vi "Extract_Channels_From_ITX.vi"(8 "error in":errorcluster, 11 "itx file, N 1d channels":path=path "P:/sample/GaAs/GaAs quantum dots/2008/PL Map/A1 735/060731ASBA_A1_6.0.itx") -> (0 "error out":errorcluster, 1 "wave names":string[](array[string]), 2 "base wavenames":string[](array[string]), 3 "Arr of 1D channels":dbl[][](array[numeric]), 4 "Notes":string)   [LabVIEW 2016]
uses:
  <userlib>/LevyLab/LV to ITX/Data.ITX/Data.ITX.lvclass
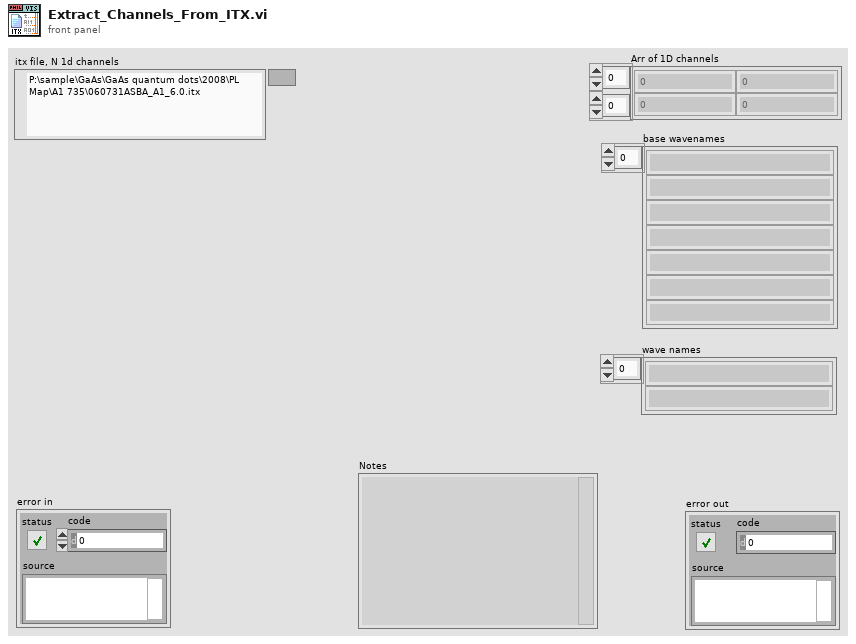
[diagram p1: front panel]
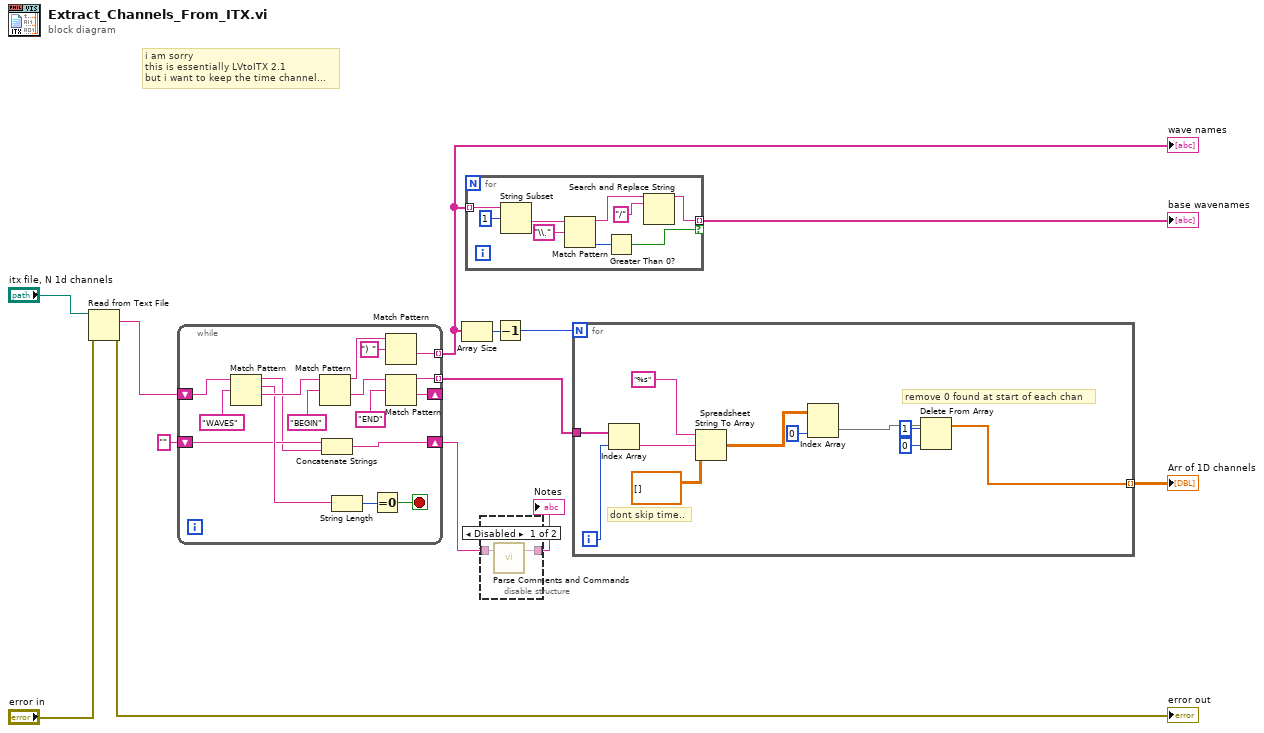
[diagram p0: block diagram]
diagram:
  # "i am sorry \nthis is essentially LVtoITX 2.1\nbut i want to keep the time channel..."
  n1 = Read from Text File(file (use dialog)="itx file, N 1d channels", error in="error in") -> (text=w6:string, error out=→"error out":errorcluster)  [unwired: 1 in, 3 out]
  n2 = while {
    tunnel: [w27] -> w12 mode=indexing
    shift-right: [w28] -> _
    shift-left: w6 -> [w15]
    tunnel: [w23] -> w8 mode=indexing
    shift-right: [w18] -> w11
    shift-left: "" ("regular expression") -> [w17]
    stop <- w24 stop-if-true
    n3 = Match Pattern(string=w15, regular expression="WAVES") -> (before substring=w16:string, match substring=w26:string, after substring=w30:string)  [unwired: 2 out]
    n4 = Match Pattern(string=w30, regular expression="BEGIN" ("regular expression 2")) -> (before substring=w14:string, after substring=w29:string)  [unwired: 3 out]
    n5 = Concatenate Strings(w17, w16) -> (w18:string)
    n6 = String Length(string=w26) -> (length=w25:i32)
    n7 = Equal To 0?(x=w25) -> (x = 0?=w24:bool)
    n8 = Match Pattern(string=w14, regular expression=") ") -> (after substring=w23:string)  [unwired: 4 out]
    n9 = Match Pattern(string=w29, regular expression="END" ("regular expression 3")) -> (before substring=w27:string, after substring=w28:string)  [unwired: 3 out]
  }
  "wave names" <- w8
  n10 = Array Size(array=w8) -> (size(s)=w9:i32)
  n11 = for {
    tunnel: w8 -> [w38] mode=indexing
    tunnel: [w31] -> w5 mode=indexing if=w34
    n12 = String Subset(string=w38, offset (0)=1) -> (substring=w37:string)  [unwired: 1 in]
    n13 = Match Pattern(string=w37, regular expression="\\.") -> (before substring=w32:string, offset past match=w35:i32)  [unwired: 1 in, 2 out]
    n14 = Greater Than 0?(x=w35) -> (x > 0?=w34:bool)
    n15 = Search and Replace String(input string=w32, search string="/") -> (result string=w31:string)  [unwired: 6 in, 3 out]
  }
  "base wavenames" <- w5
  n16 = disable-structure shown="Disabled" {
    disable-tunnel: w11 -> [w41 _]
    disable-tunnel: [w40 _] -> w10
    frame Disabled {
      n17 = call <userlib>:"Parse Comments and Commands.vi"("ITX Notes and Commands"=w41) -> ("Notes"=w40:string)  [unwired: 1 in, 1 out]
    }
    frame Enabled {
    }
  }
  "Notes" <- w10
  n18 = Decrement(x=w9) -> (x-1=w3:i32)
  n19 = for {
    N: w3 -> [_]
    tunnel: w12 -> [w52]
    tunnel: [w43] -> w4 mode=indexing
    i -> [w50]
    # "remove 0 found at start of each chan"
    # "dont skip time.."
    n20 = Index Array(array=w52, index=w50) -> (element=w51:string)
    n21 = Spreadsheet String To Array(format string="%s", spreadsheet string=w51, array type (2D Dbl)=dbl[][] []) -> (array=w48:dbl[][])  [unwired: 1 out]
    n22 = Index Array(array=w48, index (col)=0 ("disabled index (col)")) -> (element=w44:dbl[])  [unwired: 1 in]
    n23 = Delete From Array(array=w44, length=1, index=0) -> (array with subset deleted=w43:dbl[])  [unwired: 1 out]
  }
  "Arr of 1D channels" <- w4
